vi "test Get and Set Cache.vi"(8 "error in (no error)":errorcluster, 11 "TestCase in":refnum<class "Framework Property Tests.lvclass">) -> (0 "error out":errorcluster, 3 "TestCase out":refnum<class "Framework Property Tests.lvclass">)   [LabVIEW 2017, in "Framework Property Tests.lvclass"]
uses:
  Framework Property Tests.lvclass
  <vilib>/addons/_JKI Toolkits/VI Tester/TestCase.llb/TestCase.lvclass
  Classes/Transfer Group/Transfer Group.lvclass
  Classes/Transfer/Transfer.lvclass
  Classes/Framework/Framework.lvclass
  C:/Program Files (x86)/National Instruments/LabVIEW 2017/vi.lib/addons/_JKI Toolkits/VI Tester/TestCase.llb/TestCase.lvclass
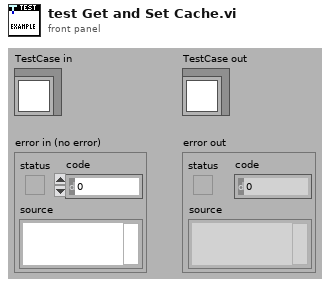
[diagram p1: front panel]
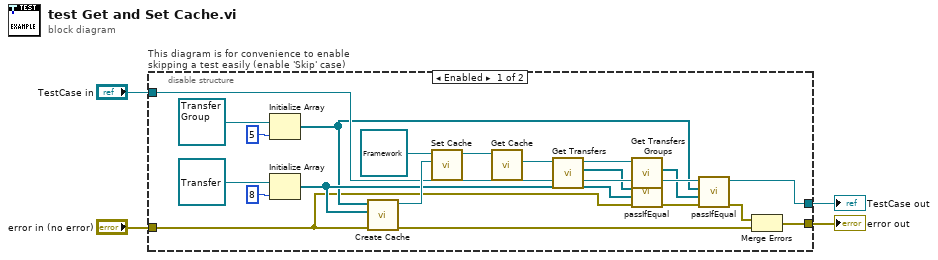
[diagram p0: block diagram]
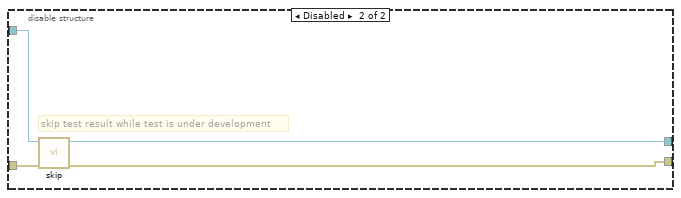
[diagram p2: hidden frame]
diagram:
  n1 = disable-structure "This diagram is for convenience to enable skipping a test easily (enable 'Skip' case)" shown="Enabled" {
    disable-tunnel: "TestCase in" -> [w17 w29]
    disable-tunnel: [w12 w27] -> w1
    disable-tunnel: [w9 w28] -> w3
    disable-tunnel: "error in (no error)" -> [w8 w26]
    frame Enabled {
      n2 = Initialize Array(refnum<class "Transfer Group.lvclass"> refnum ("DSF Core.lvlib:Transfer Group"), 5 ("dimension size")) -> (w11:refnum<class "Transfer Group.lvclass">[])
      n3 = Initialize Array(refnum<class "Transfer.lvclass"> refnum ("DSF Core.lvlib:Transfer"), 8 ("dimension size")) -> (w15:refnum<class "Transfer.lvclass">[])
      n4 = call "Create Cache.vi"("error in (no error)"=w8, "Transfers"=w15, "Transfers Groups"=w11) -> ("error out"=w5:errorcluster, "Cache out"=w20:refnum<class "Cache.lvclass">)  [unwired: 7 in]
      n5 = call "Set Cache.vi"("Cache"=w20, "Framework in"=refnum<class "Framework.lvclass"> refnum ("Mock Framework in")) -> ("Framework out"=w19:refnum<class "Framework.lvclass">)  [unwired: 9 in]
      n6 = call "Get Cache.vi"("Framework in"=w19) -> ("Cache"=w7:refnum<class "Cache.lvclass">)  [unwired: 9 in, 1 out]
      n7 = call "Get Transfers.vi"("Cache in"=w7) -> ("Transfers"=w16:refnum<class "Transfer.lvclass">[], "Cache out"=w6:refnum<class "Cache.lvclass">)  [unwired: 9 in]
      n8 = call "Get Transfers Groups.vi"("Cache in"=w6) -> ("Transfers Groups"=w10:refnum<class "Transfer Group.lvclass">[])  [unwired: 9 in, 1 out]
      n9 = call-dynamic "passIfEqual.vi"("error in (no error)"=w8, "y"=w15, "x"=w16, "TestCase in"=w17) -> ("error out"=w18:errorcluster, "TestCase out"=w13:refnum<class "Framework Property Tests.lvclass">)  [unwired: 6 in]
      n10 = call-dynamic "passIfEqual.vi"("error in (no error)"=w18, "y"=w10, "x"=w11, "TestCase in"=w13) -> ("error out"=w14:errorcluster, "TestCase out"=w12:refnum<class "Framework Property Tests.lvclass">)  [unwired: 6 in]
      n11 = Merge Errors(w14, w5) -> (w9:errorcluster)
    }
    frame Disabled {
      # "skip test result while test is under development"
      n12 = call <vilib>:"skip.vi"("error in (no error)"=w26, "TestCase in"=w29) -> ("error out"=w28:errorcluster, "TestCase out"=w27:refnum<class "Framework Property Tests.lvclass">)  [unwired: 8 in]
    }
  }
  "error out" <- w3
  "TestCase out" <- w1
